vi "softwareUpdateBase64.vi"(8 "error":errorcluster, 11 "connection ID":refnum<k5>) -> (0 "error out":errorcluster, 3 "connection ID out":refnum<k5>)   [LabVIEW 2016, in "amc_api.lvlib"]
doc: "Executes the update with base 64 file uploaded."
uses:
  amc_api.lvlib
panel:
  out "jsonRespIn":string
  out "JSON-response":string="{\"jsonrpc\":\"2.0\",\"method\":\"\",\"params\":[5,1.245,true,\"name\"],\"id\":\"1\"}"
  out "JSON request":string
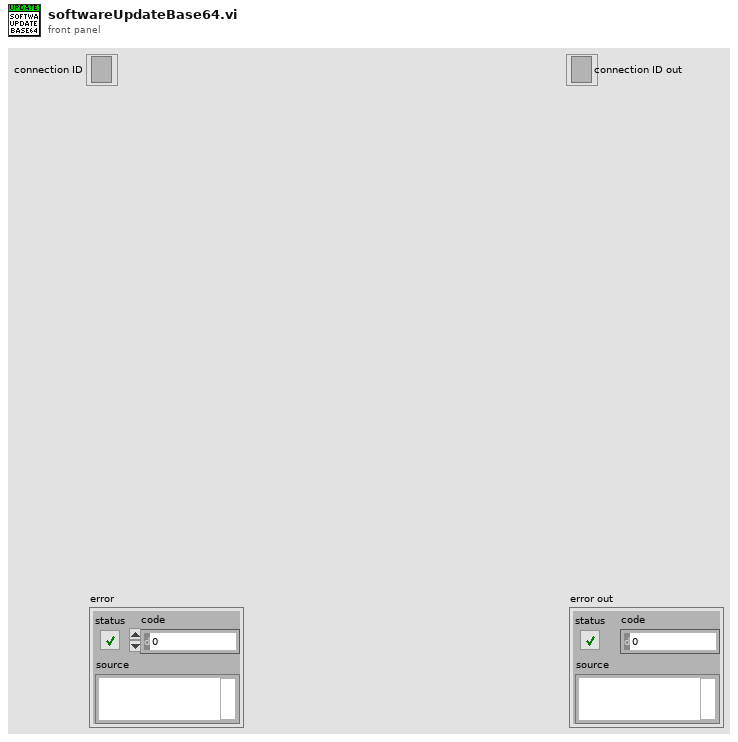
[diagram p1: front panel]
types:
  T1 = cluster{"jsonrpc":string, "method":string, "params":string[], "id":string, "api":i32, "pid":string}
  T2 = enum16{"Standard", "Buffered", "CRLF", "Immediate"}
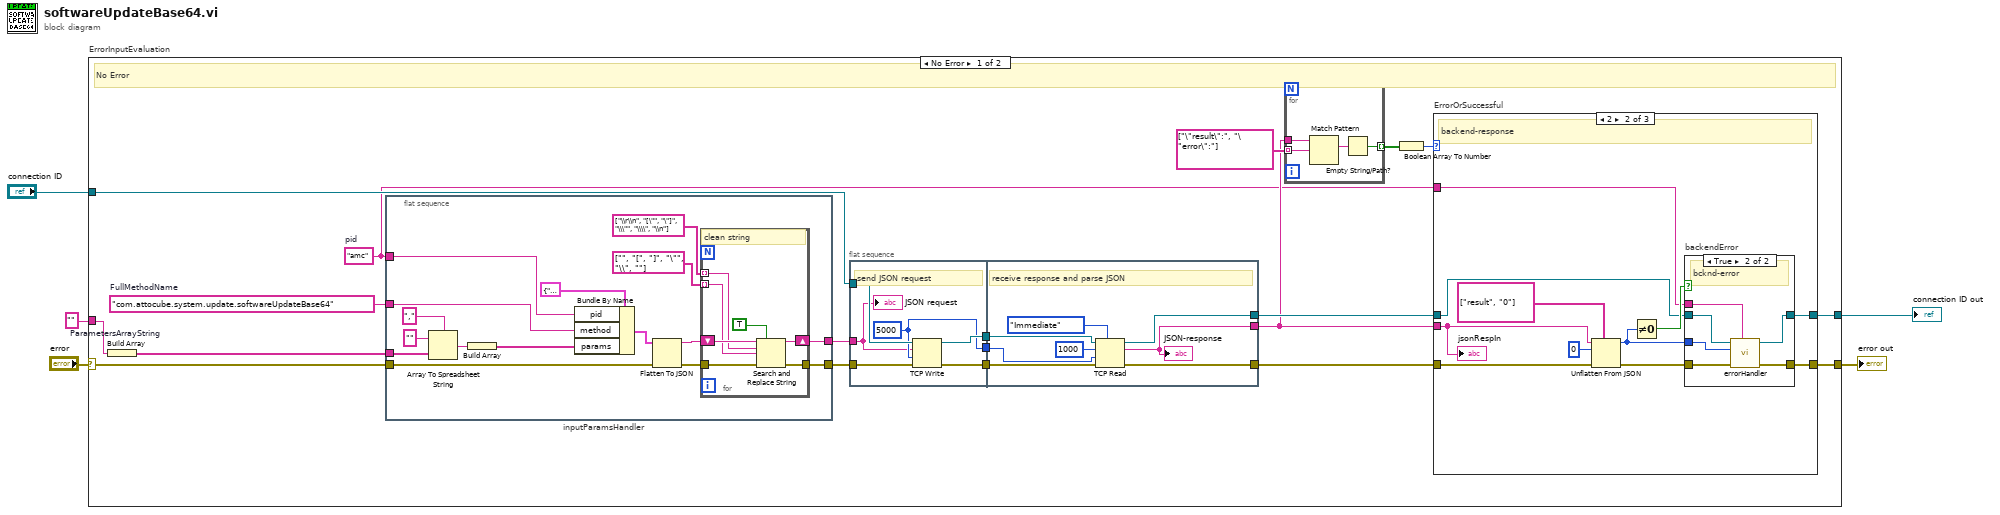
[diagram p0: block diagram]
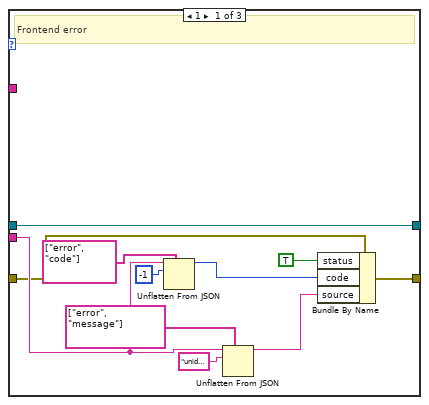
[diagram p2: hidden frame]
diagram:
  n1 = case "ErrorInputEvaluation" shown="No Error" "error" {
    selector: "error" -> [w11 w98]
    tunnel: "connection ID" -> [w21 w99]
    tunnel: [w13 w98] -> w4
    tunnel: [w14 w99] -> w3
    tunnel: "" -> [w6 _]
    frame No Error {
      w7 = "amc"  # pid
      w12 = "com.attocube.system.update.softwareUpdateBase64"  # FullMethodName
      # "No Error"
      n2 = Build Array "ParametersArrayString"(w6) -> (w10:string[])
      n3 = flat-sequence "inputParamsHandler" {
        tunnel: [w30] -> w9
        tunnel: w10 -> [w36]
        tunnel: w11 -> [w35]
        tunnel: [w32] -> w8
        tunnel: w12 -> [w26]
        tunnel: w7 -> [w25]
        frame #0 {
          n4 = Array To Spreadsheet String(delimiter (Tab)=",", array=w36, 3:"" ("format string")) -> (spreadsheet string=w38:string)
          n5 = Build Array "Build Array"(w38) -> (w27:string[])
          n6 = Bundle By Name(cluster=T1 {"jsonrpc"="2.0", "method"="com.attocube.amc.res.setRESReadOutFreq", "params"=[], "id"="1", "api"=2, "pid"=""}, "pid"=w25, "method"=w26, "params"=w27) -> (w37:T1)
          n7 = Flatten To JSON(anything=w37, error in (no error)=w35) -> (JSON string=w31:string, 11:w33:errorcluster)  [unwired: 1 in]
          n8 = for {
            tunnel: string[] ["\\r\\n", "[\"", "\"]", "\\\"", "\\\\", "\\n"] ("search string") -> [w44] mode=indexing
            tunnel: string[] ["", "[", "]", "\"", "\\", ""] ("replace string (\"\")") -> [w43] mode=indexing
            shift-right: [w46] -> w30
            shift-left: w31 -> [w45]
            tunnel: w33 -> [w42]
            tunnel: [w41] -> w32
            # "clean string"
            n9 = Search and Replace String(replace all?=TRUE ("replace all? (F)"), input string=w45, search string=w44, replace string=w43, error in=w42) -> (result string=w46:string, error out=w41:errorcluster)  [unwired: 3 in, 2 out]
          }
        }
      }
      n10 = flat-sequence {
        tunnel: w21 -> [w89]
        tunnel: [w87] -> w24
        tunnel: [w88] -> w23
        tunnel: w8 -> [w84]
        tunnel: [w86] -> w22
        tunnel: w9 -> [w85]
        tunnel: [w93] -> w17
        tunnel: w24 -> [w95]
        tunnel: w23 -> [w94]
        tunnel: [w91] -> w16
        tunnel: w22 -> [w92]
        tunnel: [w90] -> w15
        frame #0 {
          w86 = 5000 ("timeout ms (25000)")
          # "send JSON request"
          n11 = TCP Write(connection ID=w89, data in=w85, error in (no error)=w84, 9:w86) -> (connection ID out=w87:refnum<k5>, error out=w88:errorcluster)  [unwired: 1 out]
          "JSON request" <- w85
        }
        frame #1 {
          # "receive response and parse JSON"
          n12 = TCP Read(connection ID=w95, bytes to read=1000, error in (no error)=w94, 7:T2."Immediate" ("mode (standard)"), 9:w92) -> (connection ID out=w93:refnum<k5>, data out=w90:string, error out=w91:errorcluster)
          "JSON-response" <- w90
        }
      }
      n13 = for {
        tunnel: string[] ["\"result\":", "\"error\":"] ("path") -> [w50] mode=indexing
        tunnel: [w48] -> w19 mode=indexing
        tunnel: w15 -> [w51]
        n14 = Match Pattern(string=w51, regular expression=w50) -> (match substring=w49:string)  [unwired: 1 in, 3 out]
        n15 = Empty String/Path?(string/path=w49) -> (empty?=w48:bool)
      }
      n16 = Boolean Array To Number(Boolean array=w19) -> (number=w18:u32)
      n17 = case "ErrorOrSuccessful" shown="2" w18 {
        tunnel: w15 -> [w54 w64 _]
        tunnel: w17 -> [w52 w67 w83]
        tunnel: [w52 w66 w83] -> w14
        tunnel: [w55 w65 w82] -> w13
        tunnel: w16 -> [w53 w68 w82]
        tunnel: w7 -> [_ w63 _]
        frame 1 {
          # "Frontend error"
          n18 = Unflatten From JSON(path=string[] ["error", "code"], JSON string=w54, type and defaults=-1) -> (value=w61:i32)  [unwired: 4 in, 1 out]
          n19 = Unflatten From JSON(path=string[] ["error", "message"], JSON string=w54, type and defaults="unidentified error") -> (value=w62:string)  [unwired: 4 in, 1 out]
          n20 = Bundle By Name(cluster=w53, "status"=TRUE, "code"=w61, "source"=w62) -> (w55:errorcluster)
        }
        frame 2 {
          # "backend-response"
          n21 = Unflatten From JSON(path=string[] ["result", "0"], JSON string=w64, type and defaults=0, error in (no error)=w68) -> (value=w73:i32, error out=w71:errorcluster)  [unwired: 3 in]
          n22 = Not Equal To 0?(x=w73) -> (x != 0?=w72:bool)
          n23 = case "backendError" shown="True" w72 {
            tunnel: w73 -> [_ w81]
            tunnel: w71 -> [w75 w80]
            tunnel: [w74 w79] -> w66
            tunnel: [w75 w78] -> w65
            tunnel: w67 -> [w74 w77]
            tunnel: w63 -> [_ w76]
            frame False {
              # "successful"
            }
            frame True {
              # "bcknd-error"
              n24 = call "errorHandler.vi"("pid"=w76, "error in"=w80, "errNbr"=w81, "connection ID"=w77) -> ("error out 2"=w78:errorcluster, "connection ID out"=w79:refnum<k5>)  [unwired: 6 in]
            }
          }
          "jsonRespIn" <- w64
        }
        frame Default {
          # "NoResponse"
        }
      }
    }
    frame Error {
      # "Error"
    }
  }
  "error out" <- w4
  "connection ID out" <- w3
